vi "Expected message.vi"(8 "error in (no error)":errorcluster, 10 "Expected Response out":string, 11 "UI Actor in":refnum<class "UI Actor.lvclass">) -> (0 "error IO":errorcluster, 3 "UI Actor out":refnum<class "UI Actor.lvclass">)   [LabVIEW 2020, in "UI Actor.lvlib" / "UI Actor.lvclass"]
uses:
  UI Actor.lvclass
  UI Actor.lvclass/UI Actor.ctl
  Abstract/Serial Device/Serial Device.lvclass
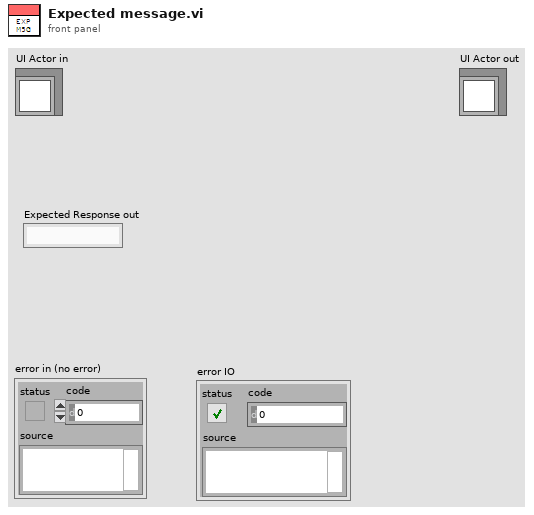
[diagram p1: front panel]
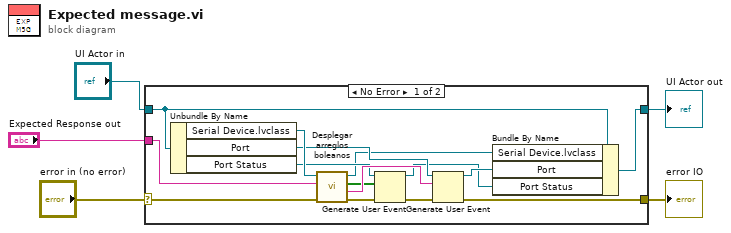
[diagram p0: block diagram]
diagram:
  n1 = case shown="No Error" "error in (no error)" {
    selector: "error in (no error)" -> [w13 w22]
    tunnel: [w12 w22] -> w1
    tunnel: [w20 w21] -> w3
    tunnel: "UI Actor in" -> [w15 w21]
    tunnel: "Expected Response out" -> [w11 _]
    frame No Error {
      n2 = Unbundle By Name(w15) -> ("Serial Device.lvclass"=w14:refnum<class "Serial Device.lvclass">, "Port"=w10:refnum<user-event>, "Port Status"=w9:refnum<user-event>)
      n3 = call-dynamic "Desplegar arreglos boleanos.vi"("error in (no error)"=w13, "Expected Response out"=w11, "Serial Device in"=w14) -> ("error out"=w18:errorcluster, "Puerto"=w17:string, "output array"=w16:bool[], "Serial Device out"=w6:refnum<class "Serial Device.lvclass">)  [unwired: 5 in]
      n4 = Generate User Event(user event=w9, event data cluster=w16, error in=w18) -> (user event out=w7:refnum<user-event>, error out=w19:errorcluster)  [unwired: 1 in]
      n5 = Generate User Event(user event=w10, event data cluster=w17, error in=w19) -> (user event out=w8:refnum<user-event>, error out=w12:errorcluster)  [unwired: 1 in]
      n6 = Bundle By Name(cluster=w15, "Serial Device.lvclass"=w6, "Port"=w8, "Port Status"=w7) -> (w20:refnum<class "UI Actor.lvclass">)
    }
    frame Error {
    }
  }
  "UI Actor out" <- w3
  "error IO" <- w1
